vi "read_params.vi"(8 "error in (no error)":errorcluster, 11 "LatentDirichletAllocation in":refnum<class "LatentDirichletAllocation.lvclass">) -> (0 "error out":errorcluster, 2 "params":T1={"n_components"=10.0, "doc_topic_prior"={"doc_topic_prior_type"="None", "doc_topic_prior_float"=0.0}, "topic_word_prior"={"topic_word_prior_type"="None", "topic_word_prior_float"=0.0}, "learning_method"="batch", "learning_decay"=0.7, "learning_offset"=10.0, "max_iter"=10.0, "batch_size"=128.0, "evaluate_every"=-1.0, "total_samples"=1000000, "perp_tol"=0.1, "mean_change_tol"=0.001, "max_doc_update_iter"=100.0, "n_jobs"=1.0, "verbose"=0.0, "random_state"=0.0}, 3 "LatentDirichletAllocation out":refnum<class "LatentDirichletAllocation.lvclass">)   [LabVIEW 2020, in "LatentDirichletAllocation.lvclass"]
uses:
  LatentDirichletAllocation.lvclass
  Controls/latent_dirichlet_allocation_params.ctl
  LatentDirichletAllocation.lvclass/LatentDirichletAllocation.ctl
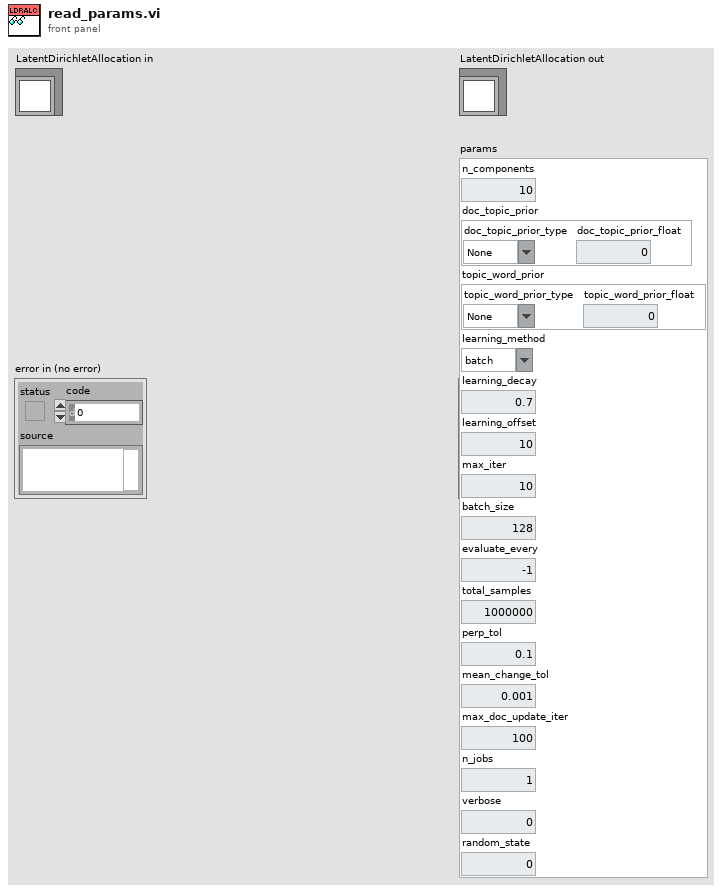
[diagram p1: front panel]
types:
  T1 = typedef "latent_dirichlet_allocation_params.ctl" = cluster{"n_components":dbl, "doc_topic_prior":cluster{"doc_topic_prior_type":string, "doc_topic_prior_float":dbl}, "topic_word_prior":cluster{"topic_word_prior_type":string, "topic_word_prior_float":dbl}, "learning_method":string, "learning_decay":dbl, "learning_offset":dbl, "max_iter":dbl, "batch_size":dbl, "evaluate_every":dbl, "total_samples":i32, "perp_tol":dbl, "mean_change_tol":dbl, "max_doc_update_iter":dbl, "n_jobs":dbl, "verbose":dbl, "random_state":dbl}
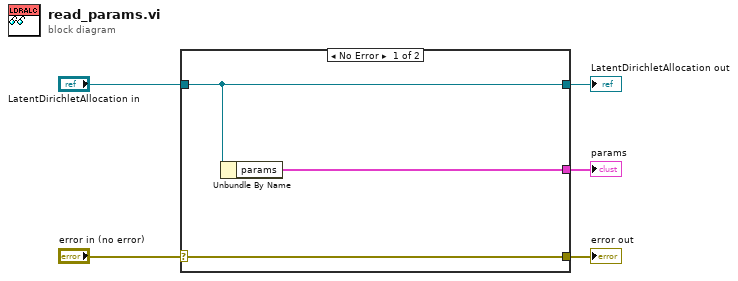
[diagram p0: block diagram]
diagram:
  n1 = case shown="No Error" "error in (no error)" {
    selector: "error in (no error)" -> [w8 w9]
    tunnel: [w8 w9] -> w4
    tunnel: [w7 w10] -> w2
    tunnel: "LatentDirichletAllocation in" -> [w7 w10]
    tunnel: [w6 _] -> w1
    frame No Error {
      n2 = Unbundle By Name(w7) -> ("params"=w6:T1)
    }
    frame Error {
    }
  }
  "error out" <- w4
  "LatentDirichletAllocation out" <- w2
  "params" <- w1
